vi "AlliGator Load Piccolo hist .bin FLI Dataset Prelude.vi"(8 "error in (no error)":errorcluster, 11 "File Path in":path) -> (0 "error out":errorcluster, 1 "Metdata":string, 2 "FLI Data File Information":T1, 3 "File Path out":path, 4 "Data Description":string)   [LabVIEW 2021, in "AlliGator Files.lvlib"]
doc: "Preliminary loading steps for Piccolo .bin files."
uses:
  AlliGator Files.lvlib
  AlliGator FLI Data File Information.ctl
  Phasor/Phasor Fluorescence Lifetime Parameters v3.ctl
  AlliGator FLI Dataset Type.ctl
  AlliGator Piccolo hist .bin Dataset Information.ctl
  AlliGator Piccolo hist BIN File Information.ctl
  AlliGator Load Single Gate Image from Piccolo hist .bin File.vi
  Phasor/Phasor.lvlib
  AlliGator HDF5.lvlib
panel:
  # "see the AlliGator License on the block diagram (Ctrl+E or Window:Show Block Diagram)"
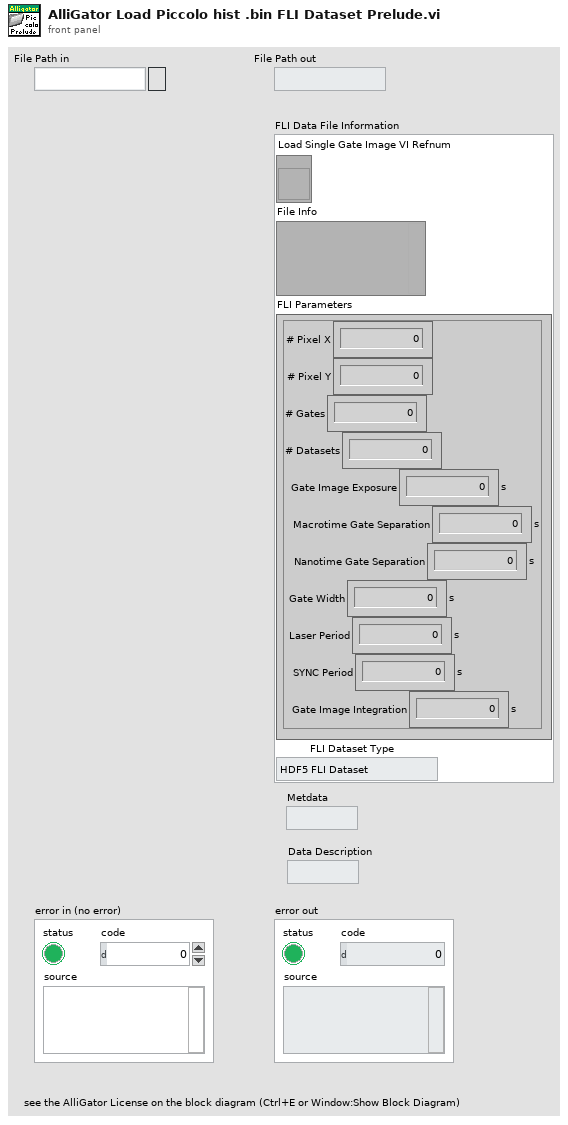
[diagram p1: front panel]
types:
  T1 = typedef "AlliGator HDF5.lvlib/AlliGator FLI Data File Information.ctl" = cluster{"Load Single Gate Image VI Refnum":refnum<vi>, "File Info":variant, "FLI Parameters":T2, "FLI Dataset Type":T3}
  T2 = typedef "Phasor.lvlib/Phasor Fluorescence Lifetime Parameters v3.ctl" = cluster{"# Pixel X":i32, "# Pixel Y":i32, "# Gates":i32, "# Datasets":i32, "Gate Image Exposure":dbl[unit], "Macrotime Gate Separation":dbl[unit], "Nanotime Gate Separation":dbl[unit], "Gate Width":dbl[unit], "Laser Period":dbl[unit], "SYNC Period":dbl[unit], "Gate Image Integration":dbl[unit]}
  T3 = typedef "AlliGator Files.lvlib/AlliGator FLI Dataset Type.ctl" = enum16{"HDF5 FLI Dataset", "Gate Image Folder", ".sdt FLI Dataset (Becker & Hickl)", ".ptu FLI Dataset (PicoQuant)", "SS1 FLI Dataset", "SS2 FLI Dataset", "I/m/phi Dataset", ".bin FLI Dataset (PicoQuant Binned)", ".bin FLI Dataset (Piccolo Binned)"}
  T4 = typedef "AlliGator Files.lvlib/AlliGator Piccolo hist .bin Dataset Information.ctl" = cluster{"File Path":path, "Piccolo hist BIN dataset Information":T5}
  T5 = typedef "AlliGator Files.lvlib/AlliGator Piccolo hist BIN File Information.ctl" = cluster{"# Pixels X":i32, "# Pixels Y":i32, "# TCSPC Bins":i32, "Temporal Resolution":dbl[unit]}
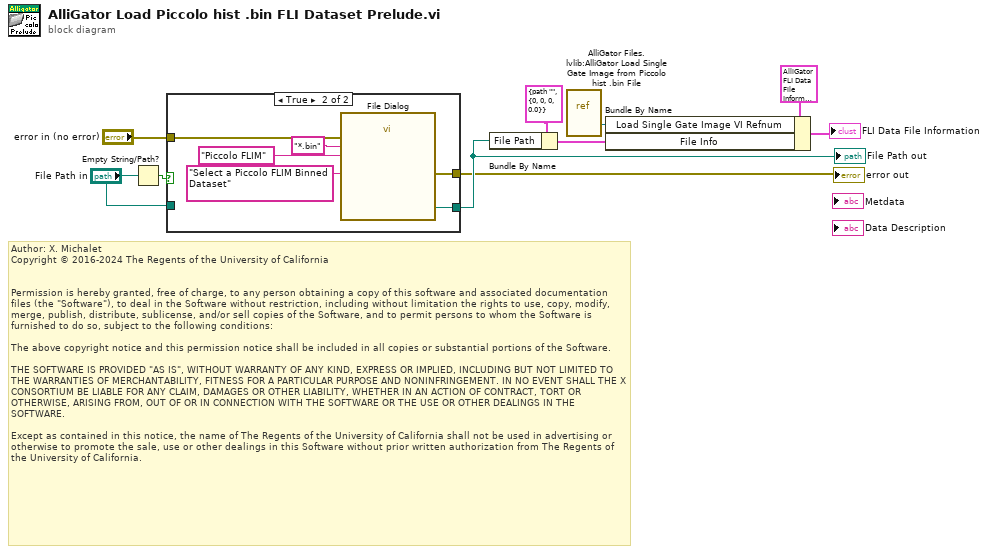
[diagram p0: block diagram]
diagram:
  # "Author: X. Michalet\nCopyright © 2016-2024 The Regents of the University of California\n \n\nPermission is hereby granted, free of charge, to any person obtaining a copy of this software and associated documentation files (the \"Software\"), to deal in the Software without restriction, including without limitation the rights to use, copy, modify, merge, publish, distribute, sublicense, and/or sell copies of the Software, and to permit persons to whom the Software is furnished to do so, subject to the following conditions:\n\nThe above copyright notice and this permission notice shall be included in all copies or substantial portions of the Software.\n\nTHE SOFTWARE IS PROVIDED \"AS IS\", WITHOUT WARRANTY OF ANY KIND, EXPRESS OR IMPLIED, INCLUDING BUT NOT LIMITED TO THE WARRANTIES OF MERCHANTABILITY, FITNESS FOR A PARTICULAR PURPOSE AND NONINFRINGEMENT. IN NO EVENT SHALL THE X CONSORTIUM BE LIABLE FOR ANY CLAIM, DAMAGES OR OTHER LIABILITY, WHETHER IN AN ACTION OF CONTRACT, TORT OR OTHERWISE, ARISING FROM, OUT OF OR IN CONNECTION WITH THE SOFTWARE OR THE USE OR OTHER DEALINGS IN THE SOFTWARE.\n\nExcept as contained in this notice, the name of The Regents of the University of California shall not be used in advertising or otherwise to promote the sale, use or other dealings in this Software without prior written authorization from The Regents of the University of California."
  n1 = Empty String/Path?(string/path="File Path in") -> (empty?=w10:bool)
  n2 = case shown="True" w10 {
    tunnel: "error in (no error)" -> [w11 w18]
    tunnel: [w12 w14] -> w4
    tunnel: [w11 w13] -> w1
    tunnel: "File Path in" -> [w12 _]
    frame False {
    }
    frame True {
      n3 = call "File Dialog"("prompt"="Select a Piccolo FLIM Binned Dataset", "error in"=w18, "pattern (all files)"="*.bin", "pattern label"="Piccolo FLIM") -> ("selected path"=w14:path, "error out"=w13:errorcluster)  [unwired: 8 in, 2 out]
    }
  }
  "error out" <- w1
  "File Path out" <- w4
  n4 = Bundle By Name(cluster=T4 {"File Path"=path "", "Piccolo hist BIN dataset Information"={"# Pixels X"=0, "# Pixels Y"=0, "# TCSPC Bins"=0, "Temporal Resolution"=0.0}} ("output cluster"), "File Path"=w4) -> (w3:T4)
  n5 = vi-ref "AlliGator Files.lvlib:AlliGator Load Single Gate Image from Piccolo hist .bin File.vi"() -> (w6:refnum<vi>)
  n6 = Bundle By Name(cluster=T1 {"Load Single Gate Image VI Refnum"=refnum, "File Info"=variant, "FLI Parameters"={"# Pixel X"=0, "# Pixel Y"=0, "# Gates"=0, "# Datasets"=0, "Gate Image Exposure"=0.0, "Macrotime Gate Separation"=0.0, "Nanotime Gate Separation"=0.0, "Gate Width"=0.0, "Laser Period"=0.0, "SYNC Period"=0.0, "Gate Image Integration"=0.0}, "FLI Dataset Type"=enum."HDF5 FLI Dataset"} ("FLI Data File Information"), "Load Single Gate Image VI Refnum"=w6, "File Info"=w3) -> (→"FLI Data File Information":T1)
